vi "Flow_Selection.vi"(7 "Offset":dbl, 9 "Linearized Temperature":sgl, 10 "Flow":dbl, 11 "Pressure Transducer 2":enum32{"Druck ", "FUJI ", "Impress"}(ring)) -> (1 "Flow rate g/s":dbl, 2 "Flow rate l/min":dbl)   [LabVIEW 2014]
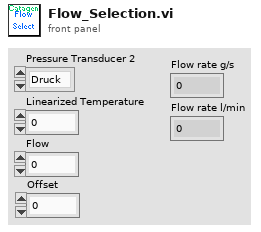
[diagram p1: front panel]
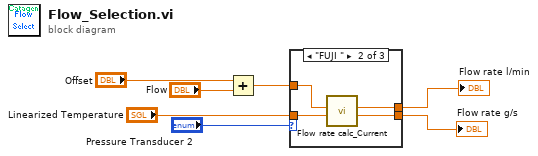
[diagram p0: block diagram]
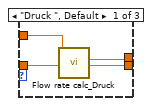
[diagram p2: hidden frame]
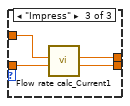
[diagram p3: hidden frame]
diagram:
  n1 = Add(x="Offset", y="Flow") -> (x+y=w1:dbl)
  n2 = case shown="\"FUJI \"" "Pressure Transducer 2" {
    tunnel: w1 -> [w11 w15 w19]
    tunnel: [w9 w13 w18] -> w5
    tunnel: "Linearized Temperature" -> [w10 w14 w17]
    tunnel: [w8 w12 w16] -> w4
    frame "Druck ", Default {
      n3 = call "Flow rate calc_Druck.vi"("T venturi"=w10, "P venturi"=w11) -> ("Flow rate g/s"=w9:dbl, "Flow rate l/min"=w8:dbl)  [unwired: 8 in]
    }
    frame "FUJI " {
      n4 = call "Flow rate calc_Current.vi"("T venturi"=w14, "P venturi"=w15) -> ("Flow rate g/s"=w13:dbl, "Flow rate l/min"=w12:dbl)  [unwired: 8 in]
    }
    frame "Impress" {
      n5 = call "Flow rate calc_Current1.vi"("T venturi"=w17, "P venturi"=w19) -> ("Flow rate g/s"=w18:dbl, "Flow rate l/min"=w16:dbl)  [unwired: 8 in]
    }
  }
  "Flow rate g/s" <- w5
  "Flow rate l/min" <- w4
